vi "Ctor.vi"(8 "error in (no error)":errorcluster, 11 "PlatformListPanel in":refnum<class "PlatformListPanel.lvclass">) -> (0 "error out":errorcluster, 3 "PlatformListPanel out":refnum<class "PlatformListPanel.lvclass">)   [LabVIEW 2020, in "PicoG-App.lvlib" / "PlatformListPanel.lvclass"]
uses:
  PlatformListPanel.lvclass
  PlatformListPanel.lvclass/PlatformListPanel.ctl
  <vilib>/IlluminatedG/IG OOPanel/OOPanel/Panel/Panel.lvclass
  <vilib>/IlluminatedG/IG OOPanel/OOPanel/ArrayManager/ArrayManager.lvclass
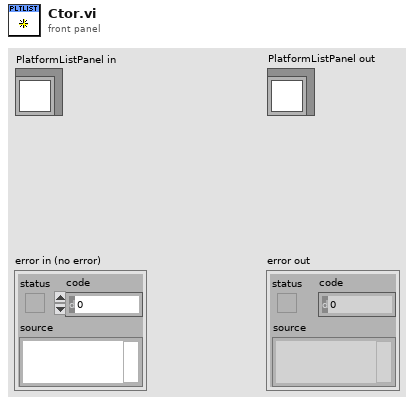
[diagram p1: front panel]
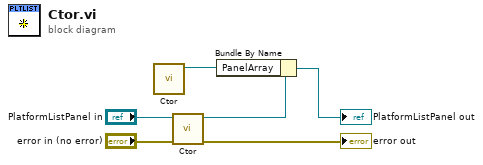
[diagram p0: block diagram]
diagram:
  n1 = call <vilib>:"Ctor.vi"() -> ("PanelArray"=w6:refnum<class "ArrayManager.lvclass">)  [unwired: 10 in, 1 out]
  n2 = call-parent <vilib>:"Ctor.vi"("error in (no error)"="error in (no error)", "Panel in"="PlatformListPanel in") -> ("error out"=→"error out":errorcluster, "Panel out"=w2:refnum<class "PlatformListPanel.lvclass">)  [unwired: 8 in]
  n3 = Bundle By Name(cluster=w2, "PanelArray"=w6) -> (→"PlatformListPanel out":refnum<class "PlatformListPanel.lvclass">)
